vi "play-AFM-CS-imaging_v2.vi"() -> ()   [LabVIEW 2017]
uses:
  z-axis-params.ctl
  controls/boolean_info.ctl
  <userlib>/_matio/level5/Public/MAT-File Data Types.ctl
  <vilib>/userdefined/High Color/nirio_resource_hc.ctl
  controls/expMetaData.ctl
  <vilib>/Utility/file.llb/Read Delimited Spreadsheet (DBL).vi
  <vilib>/FPGAPlugInAG/cRIO-9082/niLvFpga_Open_cRIO-9082.vi
  <vilib>/rvi/interface/common/dynamic/niFpgaDynamicAddResources.vi
  <vilib>/FPGAPlugInAG/Dynamic/niLvFpga_Reset_Dynamic.vi
  <vilib>/rvi/interface/common/niFpgaWaitOnOcc.vi
  <vilib>/Utility/error.llb/Error Cluster From Error Code.vi
  <vilib>/rvi/errors/niLvFpgaAdjustHostInterfaceError.vi
  <vilib>/FPGAPlugInAG/Dynamic/niLvFpga_Run_Dynamic.vi
  <vilib>/Utility/file.llb/Write Delimited Spreadsheet (DBL).vi
  <vilib>/FPGAPlugInAG/Dynamic/niLvFpga_Close_Dynamic.vi
  <userlib>/_matio/level5/Public/Write/Append Data Element.llb/Append Data Element (Anything).vi
  <vilib>/rvi/interface/nirviOpenFPGA/nirviOpenFPGA.xnode
  FPGA Bitfiles/afmimagingcontro_FPGATargetSPARTA_cs-scanningv2.lvbitx
  <vilib>/rvi/interface/nirviMethod/nirviMethod.xnode
  <vilib>/rvi/interface/nirviReadWriteControl/nirviReadWriteControl.xnode
  <vilib>/rvi/interface/nirviCloseFPGA/nirviCloseFPGA.xnode
  <vilib>/FPGAPlugInAG/Dynamic/niLvFpga_ConfigureFifo_Dynamic.vi
  <vilib>/rvi/errors/niLvFpgaMergeErrorWithErrorCode.vi
  <vilib>/rvi/interface/Simulation/niFpgaSimulationCallBeginRW.vi
  <vilib>/FPGAPlugInAG/Dynamic/niLvFpga_ReadFifo_Dynamic.vi
  fpga_interface_lib/fpga_interface.lvlib
  NiFpgaLv.dll
  <userlib>/_matio/level5.lvlib
  <vilib>/FPGAPlugInAG/Dynamic/niLvFpga_WriteFifo_Dynamic.vi
panel:
  out "xy_ref":fxp<+/-,16,5>[](array[numeric])
  out "xy_k":fxp<+/-,16,5>[](array[numeric])
  in  "input-data-path":path
  in  "Kiz_down":sgl=0.001
  in  "max_Z_settle_samples":i16=5000
  out "boolean \nindicators":T1
  out "CS Time":dbl
  out "Current Case":i16
  out "state times":dbl[](array[numeric])
  out "iter":i32
  out "entity-index":i16
  out "x = 0?":bool
  out "Numeric":i32
  out "error out 2":errorcluster
  in  "Tab Control":T2(tab)
  in  "init Z up":sgl step=0.5
  in  "trigger-0":bool
  in  "numEntities":i16
  in  "z-axis-params":T3={"TOL"=0.3, "ramp_rate"=-5e-05, "z_u_max"=5.0, "setpoint"=0.0, "Ki"=0.01, "Z_error_threshold"=0.05, "Z_settled_samples_threshold "=500, "z_UP"=1.5, "zup_N"=500, "TF Order"=1, "Num"=[1.0, 0.0, 0.0, 0.0, 0.0, 0.0, 0.0, 0.0, 0.0], "Den"=[1.0, 0.0, 0.0, 0.0, 0.0, 0.0, 0.0, 0.0, 0.0]} {"Z_error_threshold" format="%#_13g"; "ramp_rate" format="%#_4g"; "TOL" format="%#_13g"}
  in  "step_down_frac":fxp<+,8,1>=1.0
  out "output-data-path":path
  out "output-meta-data-path":path
  in  "note-blob":string
  in  "overwrite":bool
  in  "TsTicks":u32=1600
  in  "Ki-xy":sgl=0.005
  in  "collect all":bool=TRUE
  in  "collect move":bool
  in  "xy settled-samples\n threshold":i16=200
  in  "xy error-threshold":sgl=0.1
  out "number-settled-samples-x":i16
  out "number-settled-samples-y":i16
  out "case-selected":i16
  out "number-settled-samples-Z":i16
  out "size(s)":i32
  out "nsamps":i32
  out "elements left":i32=1
  out "y iter":i32
  out "size(s) 2":i32[](array[numeric])
  out "Array":i32[][](array[numeric])
  out "z-control":dbl[](graph)
  out "x-axis":dbl[](graph)
  out "z-error":dbl[](graph)
  out "y-axis":dbl[](graph)
  in  "STOP":bool
  # "- If collect all = fasle and collect move = false,\nwe only collect measurement data.\n- If collect all = false, and collect move = true,\nwe collect measurement and move data.\n- If collect all = true, we collect everything."
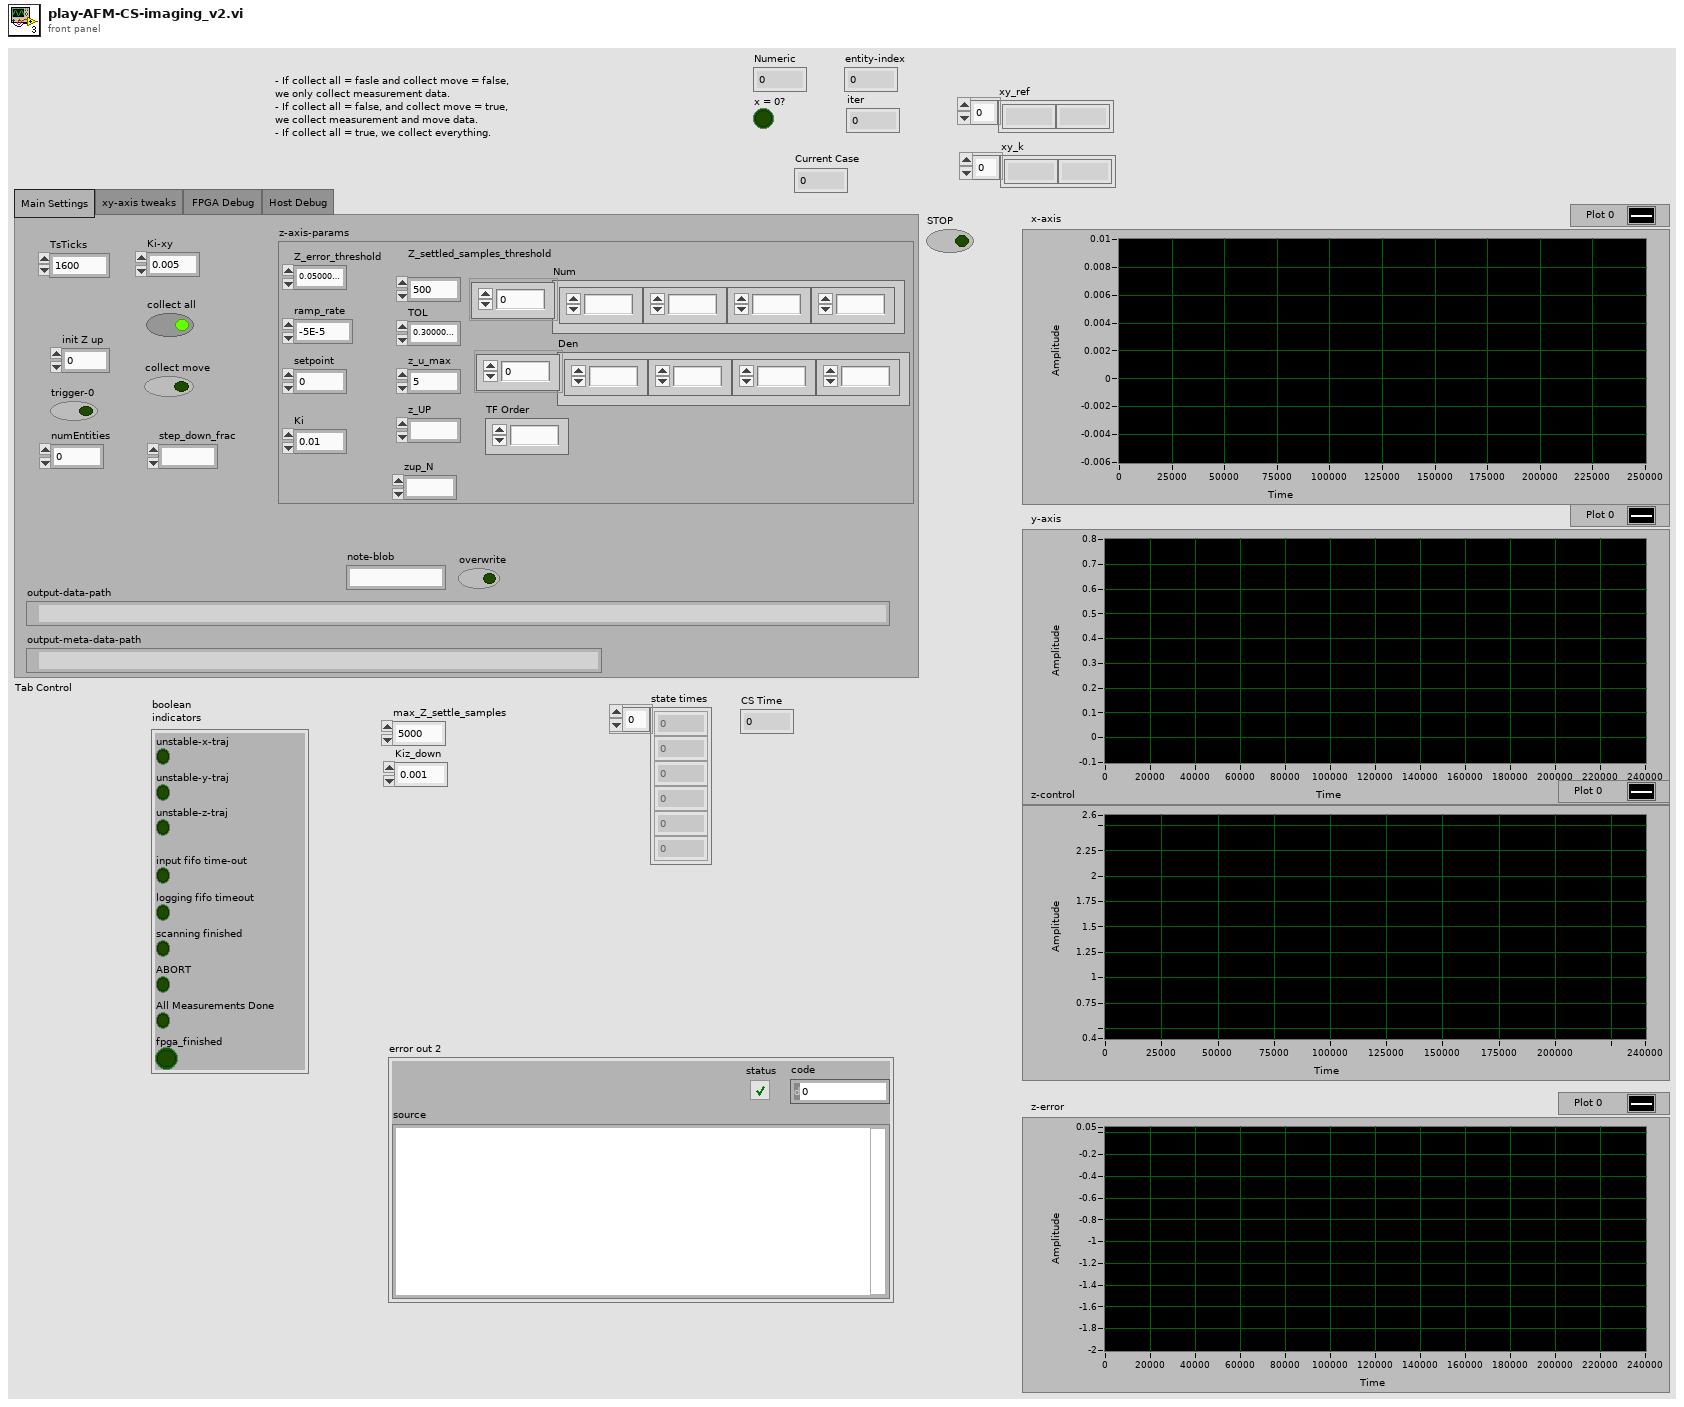
[diagram p1: front panel]
types:
  T1 = typedef "boolean_info.ctl" = cluster{"unstable-z-traj":bool, "input fifo time-out":bool, "logging fifo timeout":bool, "scanning finished":bool, "unstable-x-traj":bool, "unstable-y-traj":bool, "ABORT":bool, "All Measurements Done":bool, "fpga_finished":bool}
  T2 = enum32{"Main Settings", "xy-axis tweaks", "FPGA Debug ", "Host Debug"}
  T3 = typedef "z-axis-params.ctl" = cluster{"TOL":sgl, "ramp_rate":sgl, "z_u_max":sgl, "setpoint":sgl, "Ki":sgl, "Z_error_threshold":sgl, "Z_settled_samples_threshold ":i16, "z_UP":fxp<+/-,16,5>, "zup_N":i16, "TF Order":i32, "Num":sgl[], "Den":sgl[]}
  T4 = typedef "level5.lvlib/MAT-File Data Types.ctl" = enum32{"_invalid", "miINT8", "miUINT8", "miINT16", "miUINT16", "miINT32", "miUINT32", "miSINGLE", "_reserved_1", "miDOUBLE", "_reserved_2", "_reserved_3", "miINT64", "miUINT64", "miMATRIX", "miCOMPRESSED", "miUTF8", "miUTF16", "miUTF32"}
  T5 = typedef "nirio_resource_hc.ctl" = tag
  T6 = cluster{"unstable-z-traj":bool, "input fifo time-out":bool, "logging fifo timeout":bool, "scanning finished":bool, "unstable-x-traj":bool, "unstable-y-traj":bool, "ABORT":bool, "All Measurements Done":bool, "fpga_finished":bool}
  T7 = enum16{"open", "replace", "create", "open or create", "replace or create", "replace or create with confirmation"}
  T8 = typedef "expMetaData.ctl" = cluster{"xy_error_threshold":sgl, "xy_settled_samples_threshold":i16, "Ki_xy":sgl, "state_counts":dbl[], "TOL":sgl, "ramp_rate":sgl, "z_u_max":sgl, "setpoint":sgl, "Ki":sgl, "Z_error_threshold":sgl, "Z_settled_samples_threshold ":i16, "z_UP":sgl, "zup_N":i16, "Num":sgl[], "Den":sgl[], "max_Z_settle_samples":i16, "Kiz_down":sgl, "do_xy_CL":bool, "do_Alt_Ztrigger":bool, "output-data-path":path, "input-data-path":path, "uz_safe":sgl, "zup_rate":sgl}
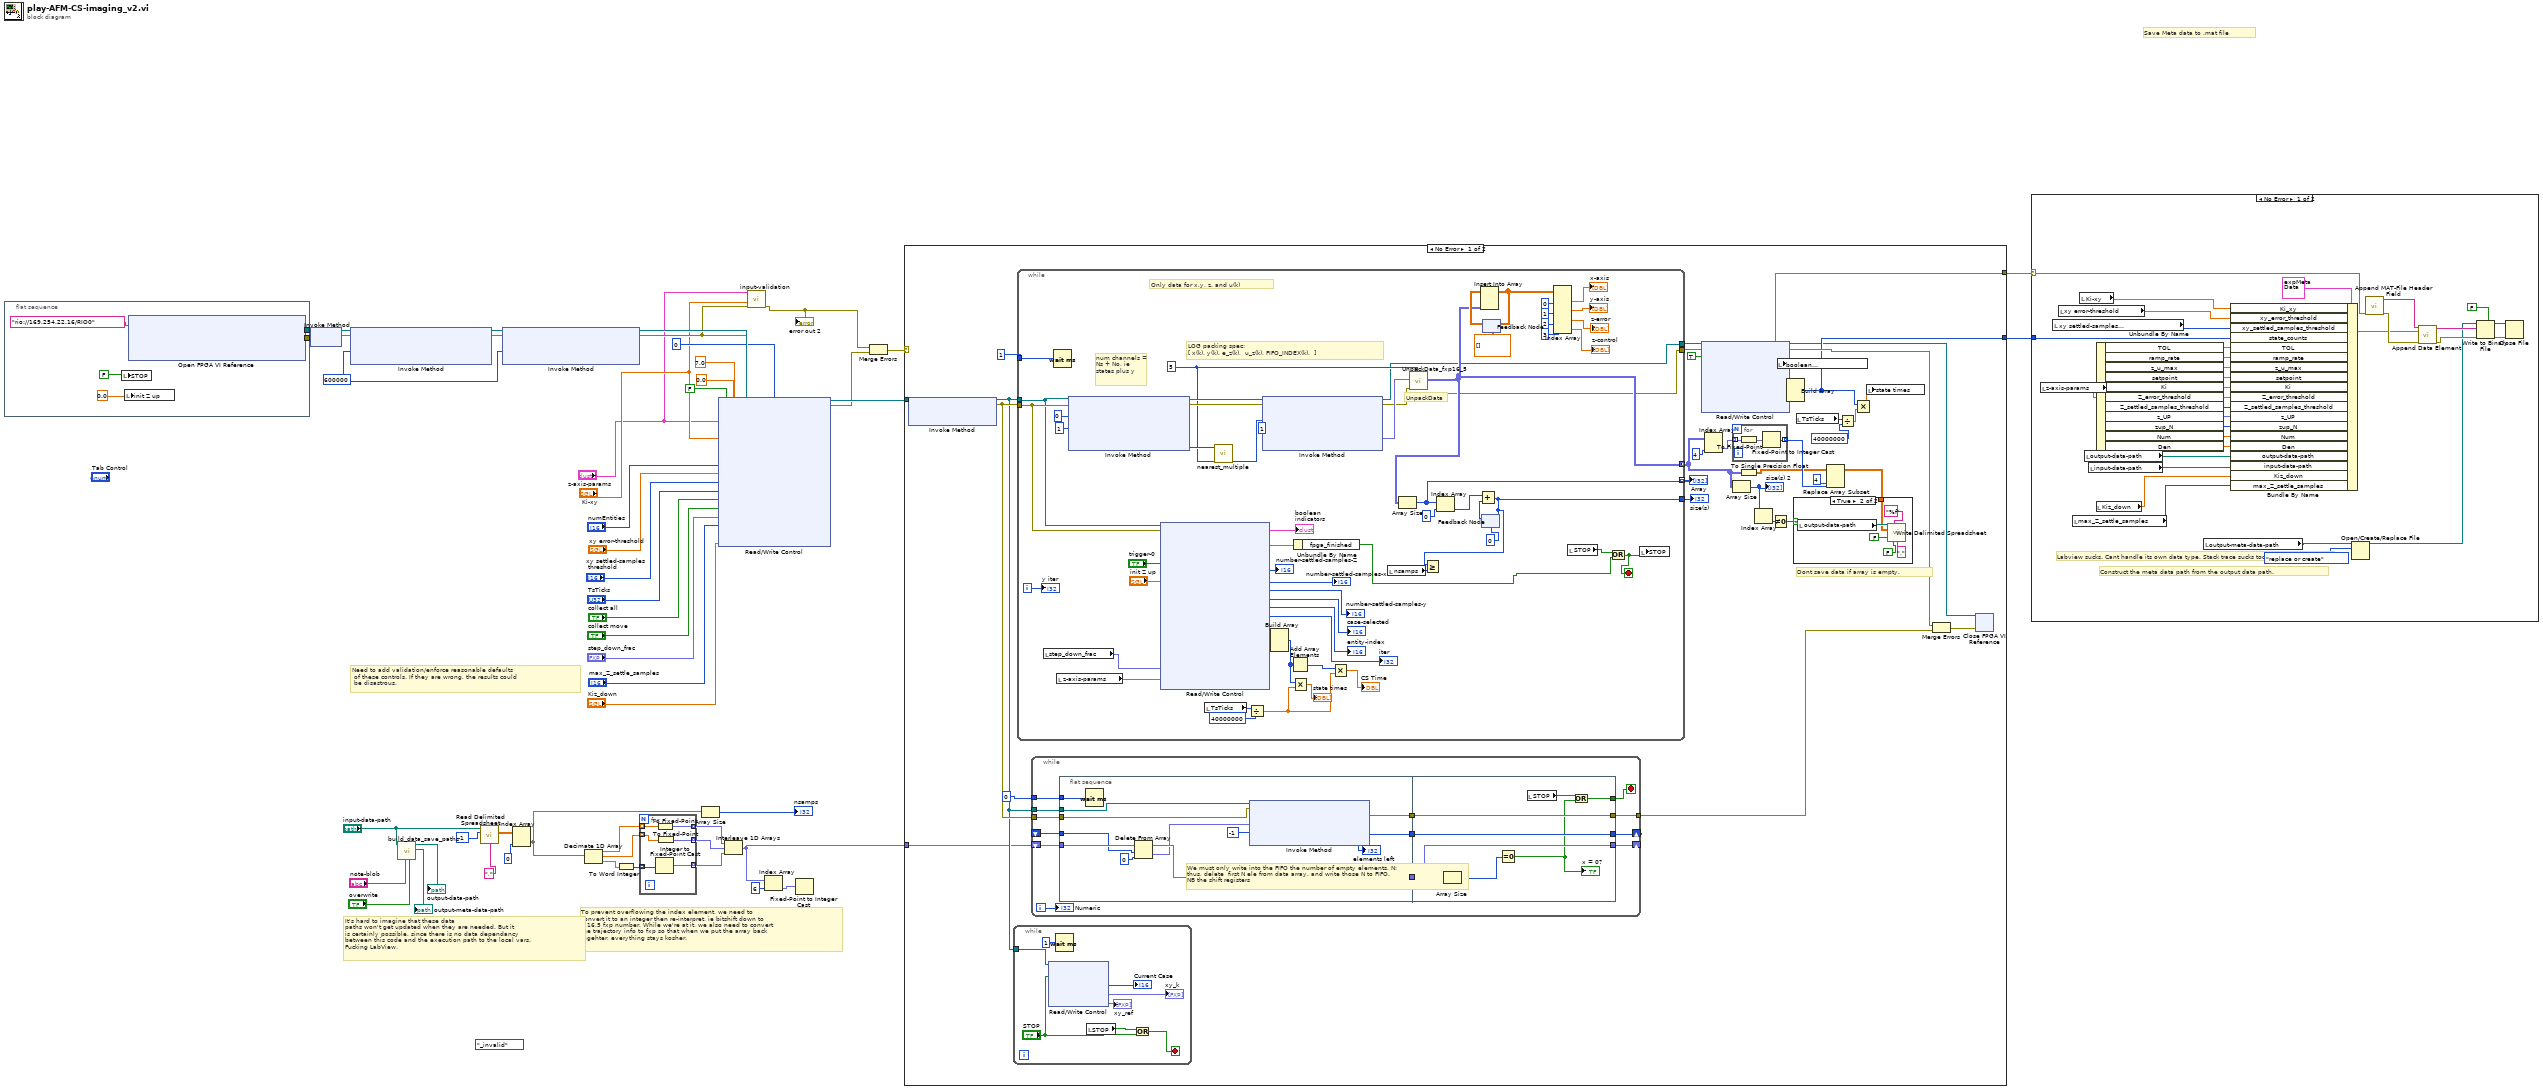
[diagram p0: block diagram]
diagram:
  (unwired) MAT-File_Data_Types."_invalid" ("MAT-File Data Types")
  w50 = 600000
  # "It's hard to imagine that these data\npaths won't get updated when they are needed. But it \nis certainly possible, since there is no data dependancy \nbetween this code and the execution path to the local vars.\nFucking LabView."
  # "Save Meta data to .mat file"
  # "To prevent overflowing the index element, we need to \nconvert it to an integer then re-interpret, ie bitshift down to \na 16,5 fxp number. While we're at it, we also need to convert\nthe trajectory info to fxp so that when we put the array back\ntogehter, everything stays kosher."
  # "Need to add validation/enforce reasonable defaults\n of these controls. If they are wrong, the results could\n be disastrous."
  n1 = flat-sequence {
    tunnel: [w56] -> w49
    tunnel: [w55] -> w48
    frame #0 {
      n2 = local write "STOP"(FALSE) -> ()
      n3 = local write "init Z up"(0.0) -> ()
      n4 = xnode "Open FPGA VI Reference"("resource name"=T5 "rio://169.254.22.16/RIO0") -> ("FPGA VI Reference Out"=w56:refnum<k20>, "error out"=w55:errorcluster)  [unwired: 1 in]
    }
  }
  n5 = xnode "Invoke Method"("FPGA VI Reference In"=w49, "error in"=w48) -> ("FPGA VI Reference Out"=w43:refnum<k20>, "error out"=w42:errorcluster)
  n6 = xnode "Invoke Method"("FPGA VI Reference In"=w43, "error in"=w42, "Requested Depth"=w50) -> ("FPGA VI Reference Out"=w45:refnum<k20>, "error out"=w46:errorcluster)  [unwired: 1 out]
  n7 = call "build_data_save_paths.vi"("overwrite"="overwrite", "note-blob"="note-blob", "input-file"="input-data-path") -> ("output-meta-data-path"=→"output-meta-data-path":path, "output-data-path"=→"output-data-path":path)  [unwired: 5 in, 2 out]
  n8 = call-poly <vilib>:"Read Delimited Spreadsheet.vi"("file path (dialog if empty)"="input-data-path", "number of rows (all:-1)"=-1, "delimiter (\\t)"=",") -> ("all rows"=w37:dbl[][])  [unwired: 7 in, 5 out]
  n9 = xnode "Invoke Method"("FPGA VI Reference In"=w45, "error in"=w46, "Requested Depth"=w50) -> ("FPGA VI Reference Out"=w51:refnum<k20>, "error out"=w29:errorcluster)  [unwired: 1 out]
  n10 = Index Array(array=w37, index (col)=0 ("dimension size")) -> (element=w15:dbl[])  [unwired: 1 in]
  n11 = Decimate 1D Array(w15) -> (w23:dbl[], w22:dbl[], w24:dbl[])
  n12 = To Word Integer(number=w24) -> (16bit integer=w21:i16[])
  n13 = for {
    tunnel: w23 -> [w62] mode=indexing
    tunnel: w22 -> [w61] mode=indexing
    tunnel: [w60] -> w19 mode=indexing
    tunnel: [w59] -> w20 mode=indexing
    tunnel: w21 -> [w58] mode=indexing
    tunnel: [w57] -> w18 mode=indexing
    n14 = Integer to Fixed-Point Cast(integer=w58) -> (fixed-point=w57:fxp<+/-,16,5>)  [unwired: 1 in]
    n15 = To Fixed-Point(number=w62) -> (fixed-point=w59:fxp<+/-,16,5>)  [unwired: 1 in]
    n16 = To Fixed-Point(number=w61) -> (fixed-point=w60:fxp<+/-,16,5>)  [unwired: 1 in]
  }
  n17 = Array Size(array=w15) -> (size(s)=→"nsamps":i32)
  n18 = xnode "Read/Write Control"("FPGA VI Reference In"=w51, "error in"=w29, "initial case"=i16 0, "z-axis-params"="z-axis-params", "xy-bound"=sgl 7.0, "Ki-xy"="Ki-xy", "init Z up"=sgl 0.0 ("u(0)"), "trigger-0"=FALSE, "numEntities"="numEntities", "xy-error-threshold"="xy error-threshold", "settled-samples threshold"="xy settled-samples\n threshold", "TsTicks"="TsTicks", "collect all"="collect all", "collect move"="collect move", "step_down_frac"="step_down_frac", "max_Z_settle_samples"="max_Z_settle_samples", "Kiz_down"="Kiz_down") -> ("FPGA VI Reference Out"=w44:refnum<k20>, "error out"=w26:errorcluster)  [unwired: 1 out]
  n19 = Interleave 1D Arrays(w20, w19, w18) -> (w14:fxp<+/-,16,5>[])
  n20 = call "input-validation.vi"("error constant"=w29, "Ki-xy"="Ki-xy", "z-axis-params"="z-axis-params") -> ("error out"=w25:errorcluster)  [unwired: 8 in]
  "error out 2" <- w25
  n21 = Index Array(array=w14, index=6) -> (element=w17:fxp<+/-,16,5>)
  n22 = Fixed-Point to Integer Cast(1:w17) -> ()  [unwired: 1 out]
  n23 = Merge Errors(w25, w26) -> (w2:errorcluster)
  n24 = case shown="No Error" w2 {
    selector: w2 -> [_ w207]
    tunnel: w44 -> [w97 _]
    tunnel: w14 -> [w95 _]
    tunnel: [w94 w207] -> w11
    tunnel: [w93 _] -> w10
    frame No Error {
      # "Dont save data if array is empty."
      n25 = xnode "Invoke Method"("FPGA VI Reference In"=w97) -> ("FPGA VI Reference Out"=w96:refnum<k20>, "error out"=w98:errorcluster)  [unwired: 2 in]
      n26 = while {
        tunnel: w96 -> [w115]
        stop <- w111 stop-if-true
        n27 = xnode "Read/Write Control"("FPGA VI Reference In"=w115, "ABORT"="STOP") -> ("Current Case"=→"Current Case":u8, "xy_k"=→"xy_k":fxp<+/-,16,5>[], "xy_ref"=→"xy_ref":fxp<+/-,16,5>[])  [unwired: 1 in, 2 out]
        n28 = Wait (ms)(milliseconds to wait=u32 1) -> ()  [unwired: 1 out]
        n29 = local read "STOP"() -> (w112:bool)
        n30 = Or(x=w112, y="STOP") -> (x .or. y?=w111:bool)
      }
      n31 = while {
        tunnel: 1 -> [w206]
        tunnel: w96 -> [w194]
        tunnel: w98 -> [w195]
        tunnel: [w159] -> w87
        tunnel: [w170] -> w78 mode=concatenating
        tunnel: [w192] -> w91
        tunnel: [w168] -> w86
        tunnel: [w185] -> w83 mode=indexing
        i -> [w193]
        stop <- w186 stop-if-true
        w171 = u32 5 ("y")
        # "LOG packing spec:\n[ x(k), y(k), e_z(k),  u_z(k), FIFO_INDEX(k),  ]"
        # "num channels = Ns + No, ie states plus y"
        # "Only data for x,y, z, and u(k)"
        # "UnpackData"
        n32 = local read "step_down_frac"() -> (w147:fxp<+,8,1>)
        n33 = Wait (ms)(milliseconds to wait=w206) -> ()  [unwired: 1 out]
        n34 = local read "z-axis-params"() -> (w148:T3)
        n35 = xnode "Invoke Method"("FPGA VI Reference In"=w194, "error in"=w195, "Number of Elements"=0 ("Timeout (ms)"), "Timeout (ms)"=1) -> ("FPGA VI Reference Out"=w202:refnum<k20>, "error out"=w203:errorcluster, "Elements Remaining"=w189:u32)  [unwired: 1 out]
        n36 = xnode "Read/Write Control"("FPGA VI Reference In"=w194, "error in"=w195, "trigger-0"="trigger-0", "init Z up"="init Z up", "step_down_frac"=w147, "z-axis-params"=w148) -> ("boolean  indicators"=w152:T6, "number-settled-samples-Z"=→"number-settled-samples-Z":i16, "number-settled-samples-x"=→"number-settled-samples-x":i16, "number-settled-samples-y"=→"number-settled-samples-y":i16, "Current Case"=→"case-selected":u8, "entity-index"=→"entity-index":i16, "iter"=→"iter":i32, "state1-count"=w164:u64, "state2-count"=w163:u64, "state3-count"=w162:u64, "state4-count"=w161:u64, "state5-count"=w160:u64)  [unwired: 1 in, 3 out]
        "boolean \nindicators" <- w152
        n37 = local read "TsTicks"() -> (w155:u32)
        n38 = call "nearest_multiple.vi"("numChan"=w171, "N"=w189) -> ("(int) y*floor(x/y)"=w188:u64)  [unwired: 9 in]
        n39 = Divide(x=w155, y=u32 40000000) -> (x/y=w150:dbl)
        n40 = xnode "Invoke Method"("FPGA VI Reference In"=w202, "error in"=w203, "Number of Elements"=w188, "Timeout (ms)"=1) -> ("FPGA VI Reference Out"=w159:refnum<k20>, "error out"=w168:errorcluster, "Data"=w169:fxp<+/-,16,5>[])  [unwired: 1 out]
        n41 = Build Array(w164, w163, w162, w161, w160) -> (w151:u64[])
        n42 = Add Array Elements(numeric array=w151) -> (sum=w156:u64)
        n43 = Multiply(x=w151, y=w150) -> (x*y=→"state times":dbl[])
        n44 = Unbundle By Name(w152) -> ("fpga_finished"=w167:bool)
        n45 = Multiply(x=w156, y=w150) -> (x*y=→"CS Time":dbl)
        n46 = local read "nsamps"() -> (w199:i32)
        n47 = call "UnpackData_fxp16_5.vi"("NumChannels"=w171, "error In"=w168, "1D Data In"=w169) -> ("2D Data Out"=w170:fxp<+/-,16,5>[][])  [unwired: 7 in, 1 out]
        n48 = Array Size(array=w170) -> (size(s)=w185:i32[])
        n49 = Index Array(array=w185, index=0) -> (element=w197:i32)
        n50 = feedback #1(0) -> (w198:i32)
        n51 = Add(x=w197, y=w198) -> (x+y=w192:i32)
        n52 = Greater Or Equal?(x=w192, y=w199) -> ()  [unwired: 1 out]
        n53 = feedback-in #1(w192) -> ()
        n54 = feedback #2(dbl[][] []) -> (w181:dbl[][])
        n55 = Insert Into Array(array=w181, new element=w170) -> (w172:dbl[][])  [unwired: 2 in]
        n56 = feedback-in #2(w172) -> ()
        n57 = Index Array(array=w172, index (col) #1=0 ("disabled index (col)"), index (col) #2=1 ("index (col)"), index (col) #3=2 ("index (col)"), index (col) #4=3 ("index (col)")) -> (element #1=→"x-axis":dbl[], element #2=→"y-axis":dbl[], element #3=→"z-error":dbl[], element #4=→"z-control":dbl[])  [unwired: 4 in]
        n58 = local read "STOP"() -> (w187:bool)
        n59 = Or(x=w187, y=w167) -> (x .or. y?=w186:bool)
        n60 = local write "STOP"(w186) -> ()
        "y iter" <- w193
      }
      "size(s)" <- w91
      "Array" <- w83
      n61 = while {
        tunnel: [w126] -> w88
        tunnel: 0 -> [w128]
        shift-right: [w122] -> _
        shift-left: _ -> [w125]
        shift-right: [w120] -> _
        shift-left: w95 -> [w127]
        tunnel: w96 -> [w119]
        tunnel: w98 -> [w118]
        i -> [w116]
        stop <- w117 stop-if-true
        n62 = flat-sequence {
          tunnel: w128 -> [w139]
          tunnel: w127 -> [w134]
          tunnel: w125 -> [w130]
          tunnel: [w137] -> w124
          tunnel: [w135] -> w123
          tunnel: [w136] -> w121
          tunnel: w119 -> [w132]
          tunnel: w118 -> [w131]
          tunnel: [w146] -> w122
          tunnel: [w143] -> w126
          tunnel: w124 -> [w143]
          tunnel: w123 -> [w146]
          tunnel: w121 -> [w144]
          tunnel: [w144] -> w120
          tunnel: [w140] -> w117
          frame #0 {
            # "We must only write into the FIFO the number of empty elements, N:\nthus, delete  first N ele from data array, and write those N to FIFO.\nNB the shift registers"
            n63 = Wait (ms)(milliseconds to wait=w139) -> ()  [unwired: 1 out]
            n64 = Delete From Array(array=w134, length=w130, index=0) -> (deleted portion=w133:fxp<+/-,16,5>[], array with subset deleted=w136:fxp<+/-,16,5>[])
            n65 = xnode "Invoke Method"("FPGA VI Reference In"=w132, "error in"=w131, "Data"=w133, "Timeout (ms)"=-1) -> ("error out"=w137:errorcluster, "Empty Elements Remaining"=w135:u32)  [unwired: 1 out]
            "elements left" <- w135
          }
          frame #1 {
            n66 = Array Size(array=w144) -> (size(s)=w145:i32)
            n67 = Equal To 0?(x=w145) -> (x = 0?=w142:bool)
            "x = 0?" <- w142
            n68 = local read "STOP"() -> (w141:bool)
            n69 = Or(x=w141, y=w142) -> (x .or. y?=w140:bool)
          }
        }
        "Numeric" <- w116
      }
      n70 = xnode "Read/Write Control"("FPGA VI Reference In"=w87, "error in"=w86, "ABORT"=TRUE) -> ("FPGA VI Reference Out"=w84:refnum<k20>, "error out"=w94:errorcluster, "boolean  indicators"=w67:T6, "state1-count"=w76:u64, "state2-count"=w75:u64, "state3-count"=w74:u64, "state4-count"=w73:u64, "state5-count"=w72:u64)
      n71 = Index Array(array=w78, index (col)=4) -> (element=w81:fxp<+/-,16,5>[])  [unwired: 1 in]
      n72 = for {
        tunnel: w81 -> [w106] mode=indexing
        tunnel: [w107] -> w79 mode=indexing
        n73 = To Fixed-Point(number=w106) -> (fixed-point=w105:fxp<+/-,16,5>)  [unwired: 1 in]
        n74 = Fixed-Point to Integer Cast(1:w105) -> (0:w107:i16)
      }
      n75 = Array Size(array=w78) -> (size(s)=w68:i32[])
      "size(s) 2" <- w68
      n76 = To Single Precision Float(number=w78) -> (single precision float=w77:sgl[][])
      n77 = Index Array(array=w68) -> (element=w69:i32)  [unwired: 1 in]
      n78 = Not Equal To 0?(x=w69) -> (x != 0?=w70:bool)
      n79 = local write "boolean \nindicators"(w67) -> ()
      n80 = Build Array(w76, w75, w74, w73, w72) -> (w93:u64[])
      n81 = local read "TsTicks"() -> (w66:u32)
      n82 = Replace Array Subset(array=w77, new element=w79, index (col)=4) -> (w71:sgl[][])  [unwired: 1 in]
      n83 = case shown="True" w70 {
        tunnel: w71 -> [_ w99]
        frame False {
        }
        frame True {
          n84 = local read "output-data-path"() -> (w104:path)
          n85 = call-poly <vilib>:"Write Delimited Spreadsheet.vi"("file path (dialog if empty)"=w104, "format (%.3f)"="%f", "2D data"=w99, "append to file? (new file:F)"=FALSE, "transpose? (no:F)"=FALSE, "delimiter (\\t)"=",") -> ()  [unwired: 8 in, 2 out]
        }
      }
      n86 = Divide(x=w66, y=u32 40000000) -> (x/y=w64:dbl)
      n87 = Multiply(x=w93, y=w64) -> (x*y=w63:dbl[])
      n88 = local write "state times"(w63) -> ()
      n89 = Merge Errors(w94, w88) -> (w89:errorcluster)
      n90 = xnode "Close FPGA VI Reference"("FPGA VI Reference In"=w84, "error in"=w89) -> ()  [unwired: 1 out]
    }
    frame Error {
    }
  }
  n91 = case shown="No Error" w11 {
    selector: w11 -> [w233 _]
    tunnel: w10 -> [w220 _]
    frame No Error {
      # "Construct the meta data path from the output data path."
      # "Labview sucks. Cant handle its own data type. Stack trace sucks too."
      n92 = local read "z-axis-params"() -> (w219:T3)
      n93 = local read "xy settled-samples\n threshold"() -> (w216:i16)
      n94 = local read "xy error-threshold"() -> (w217:sgl)
      n95 = local read "max_Z_settle_samples"() -> (w209:i16)
      n96 = local read "Ki-xy"() -> (w218:sgl)
      n97 = local read "output-data-path"() -> (w211:path)
      n98 = local read "input-data-path"() -> (w210:path)
      n99 = Unbundle By Name(w219) -> ("TOL"=w230:sgl, "ramp_rate"=w229:sgl, "z_u_max"=w228:sgl, "setpoint"=w227:sgl, "Ki"=w226:sgl, "Z_error_threshold"=w225:sgl, "Z_settled_samples_threshold"=w224:i16, "z_UP"=w223:fxp<+/-,16,5>, "zup_N"=w222:i16, "Num"=w213:sgl[], "Den"=w212:sgl[])
      n100 = local read "Kiz_down"() -> (w208:sgl)
      n101 = local read "output-meta-data-path"() -> (w214:path)
      n102 = Bundle By Name(cluster=T8 {"xy_error_threshold"=0.1, "xy_settled_samples_threshold"=200, "Ki_xy"=0.005, "state_counts"=[], "TOL"=0.3, "ramp_rate"=-5e-06, "z_u_max"=5.0, "setpoint"=0.0, "Ki"=0.001, "Z_error_threshold"=0.0, "Z_settled_samples_threshold "=0, "z_UP"=1.5, "zup_N"=5000, "Num"=[-0.00254, 0.000408, 0.00295, 0.0, 0.0, 0.0, 0.0, 0.0, 0.0], "Den"=[0.982758, -1.98194, 1.0, 0.0, 0.0, 0.0, 0.0, 0.0, 0.0], "max_Z_settle_samples"=5000, "Kiz_down"=0.001, "do_xy_CL"=FALSE, "do_Alt_Ztrigger"=FALSE, "output-data-path"=path "", "input-data-path"=path "", "uz_safe"=0.0, "zup_rate"=0.0} ("ExpMetaData"), "Ki_xy"=w218, "xy_error_threshold"=w217, "xy_settled_samples_threshold"=w216, "state_counts"=w220, "TOL"=w230, "ramp_rate"=w229, "z_u_max"=w228, "setpoint"=w227, "Ki"=w226, "Z_error_threshold"=w225, "Z_settled_samples_threshold"=w224, "z_UP"=w223, "zup_N"=w222, "Num"=w213, "Den"=w212, "output-data-path"=w211, "input-data-path"=w210, "Kiz_down"=w208, "max_Z_settle_samples"=w209) -> (w231:T8)
      n103 = Open/Create/Replace File(file path (use dialog)=w214, operation (0:open)=T7."replace or create") -> (refnum out=w232:refnum<file>)  [unwired: 4 in, 2 out]
      n104 = call <userlib>:"Append MAT-File Header Field.vi"("error"=w233) -> ("result string"=w240:string, "error out"=w234:errorcluster)  [unwired: 13 in]
      n105 = call-poly <userlib>:"Append Data Element.vi"("initial string"=w240, "data"=w231, "error in (no error)"=w234) -> ("result string"=w238:string, "error out"=w239:errorcluster)  [unwired: 11 in]
      n106 = Write to Binary File(file (use dialog)=w232, data=w238, error in=w239, 5:FALSE ("prepend array or string size? (T)")) -> (refnum out=w235:refnum<file>, error out=w236:errorcluster)  [unwired: 2 in, 1 out]
      n107 = Close File(refnum=w235, error in=w236) -> ()  [unwired: 2 out]
    }
    frame Error {
    }
  }
